vi "GetChannelImpedance.vi"(8 "error in (no error)":errorcluster, 11 "TektronixDPO_PhysicalDevice.lvclass":refnum<class "TektronixDPO_PhysicalDevice.lvclass">) -> (0 "error out":errorcluster, 3 "TektronixDPO_PhysicalDevice.lvclassOut":refnum<class "TektronixDPO_PhysicalDevice.lvclass">)   [LabVIEW 2013, in "TektronixDPO_PhysicalDevice.lvclass"]
doc: "Read from the phsyical device the offset relative to the specified channel"
uses:
  TektronixDPO_PhysicalDevice.lvclass
  shared/Typdefs/Choice78.ctl
  TektronixDPO_PhysicalDevice.lvclass/TektronixDPO_PhysicalDevice.ctl
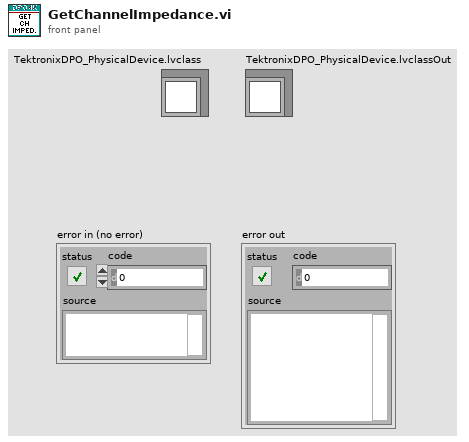
[diagram p1: front panel]
types:
  T1 = typedef "Choice78.ctl" = enum16{"1M", "75", "50"}
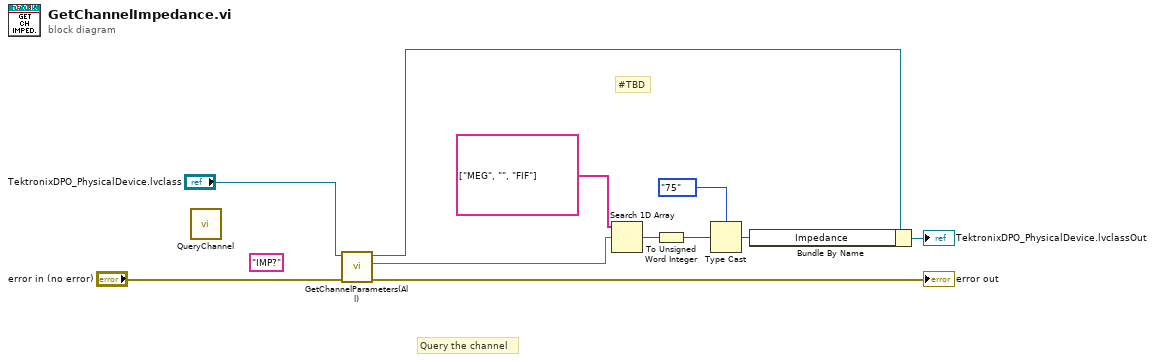
[diagram p0: block diagram]
diagram:
  (unwired) "IMP?" ("string")
  # "#TBD"
  # "Query the channel"
  n1 = call "QueryChannel.vi"() -> ()  [unwired: 10 in, 2 out]
  n2 = call "GetChannelParameters(All).vi"("error in (no error)"="error in (no error)", "TektronixDPO_PhysicalDevice in"="TektronixDPO_PhysicalDevice.lvclass") -> ("error out"=→"error out":errorcluster, "Response"=w3:string, "TektronixDPO_PhysicalDevice out"=w8:refnum<class "TektronixDPO_PhysicalDevice.lvclass">)  [unwired: 7 in]
  n3 = Search 1D Array(1D array=string[] ["MEG", "", "FIF"], element=w3) -> (index of element=w4:i32)  [unwired: 1 in]
  n4 = To Unsigned Word Integer(number=w4) -> (unsigned 16bit integer=w5:u16)
  n5 = Type Cast(type=Choice78."75" ("Channel0"), x=w5) -> (*(type *) &x=w1:T1)
  n6 = Bundle By Name(cluster=w8, "Impedance"=w1) -> (→"TektronixDPO_PhysicalDevice.lvclassOut":refnum<class "TektronixDPO_PhysicalDevice.lvclass">)
